vi "Check INI Settings.vi"(8 "error in (no error)":errorcluster) -> (0 "error out":errorcluster, 1 "found?":bool, 2 "value":bool)   [LabVIEW 2013, in "SET Project Editor.lvlib"]
doc: "Check INI Settings.vi\n\nCheck \"LabVIEW.ini\" for \"UseUnicode\". Outputs:\nfound? = True if \"UseUnicode\" is found\nvalue = Value of \"UseUnicode\" entry"
uses:
  SET Project Editor.lvlib
  <vilib>/Utility/config.llb/Read Key (Boolean).vi
  <vilib>/Utility/config.llb/NI_LVConfig.lvlib
panel:
  # "Check INI Settings.vi\n\nCheck \"LabVIEW.ini\" for \"UseUnicode\". Outputs:\nfound? = True if \"UseUnicode\" is found\nvalue = Value of \"UseUnicode\" entry"
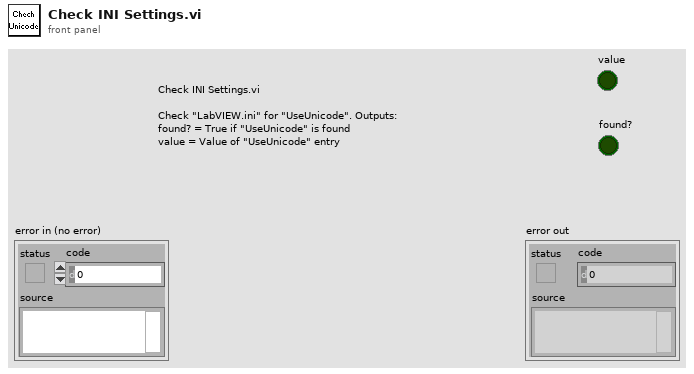
[diagram p1: front panel]
types:
  T1 = typedef "NI_LVConfig.lvlib/Config Data RefNum.ctl" = refnum<k1>
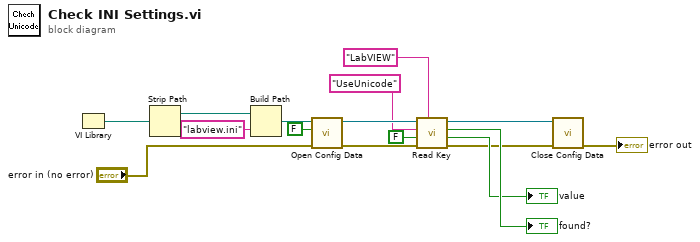
[diagram p0: block diagram]
diagram:
  n1 = VI Library() -> (path=w16:path)
  n2 = Strip Path(path=w16) -> (stripped path=w15:path)  [unwired: 1 out]
  n3 = Build Path(base path=w15, name or relative path="labview.ini") -> (appended path=w13:path)
  n4 = call <vilib>:"Open Config Data.vi"("error in (no error)"="error in (no error)", "create file if necessary (T)"=FALSE, "configuration file path"=w13) -> ("error out"=w10:errorcluster, "refnum"=w11:T1)  [unwired: 6 in, 1 out]
  n5 = call-poly <vilib>:"Read Key.vi"("section"="LabVIEW", "error in (no error)"=w10, "default value"=FALSE, "key"="UseUnicode", "refnum"=w11) -> ("error out"=w5:errorcluster, "value"=→"value":bool, "found?"=→"found?":bool, "refnum out"=w6:T1)  [unwired: 3 in]
  n6 = call <vilib>:"Close Config Data.vi"("error in (no error)"=w5, "refnum"=w6) -> ("error out"=→"error out":errorcluster)  [unwired: 8 in, 1 out]
